vi "GetStartAndStopBlocks.vi"(8 "error in (no error)":errorcluster, 9 "data":T1) -> (0 "error out":errorcluster, 2 "stop block":T5, 3 "start block":T5)   [LabVIEW 2017, in "CmsDataEventCreator.lvlib"]
uses:
  <vilib>/addons/InsightCM/Devices/Shared/Cms/CmsDataEventCreator/CmsDataEventCreator.lvlib
  <vilib>/addons/InsightCM/Devices/Shared/Common/DVRBuffer/controls/BufferLocation.ctl
  <vilib>/addons/InsightCM/Devices/Shared/Common/DataFlow/controls/Data.ctl
  <vilib>/addons/InsightCM/Utilities/DataAccessors/controls/wfmSGL_DVR.ctl
  <vilib>/addons/PointValueMap/controls/PointMap.ctl
  <vilib>/addons/InsightCM/Devices/Shared/Common/DataFlow/controls/Type.ctl
  <vilib>/addons/PointValueMap/subVIs/Point_Read_variant.vi
  <vilib>/addons/PointValueMap/PointValueMap.lvlib
  <vilib>/addons/InsightCM/Devices/Shared/Common/DVRBuffer/DVRBuffer.lvlib
  <vilib>/addons/InsightCM/Devices/Shared/Common/DataFlow/DataFlow.lvlib
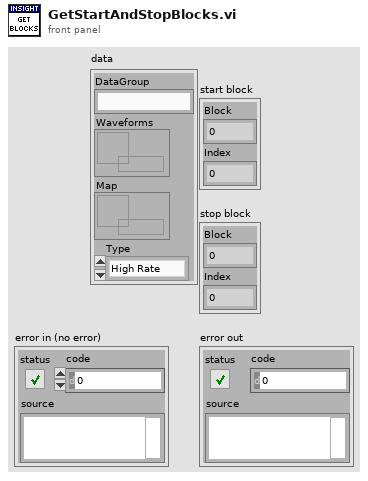
[diagram p1: front panel]
types:
  T1 = typedef "DataFlow.lvlib/Data.ctl" = cluster{"DataGroup":string, "Waveforms":T2, "Map":T3, "Type":T4}
  T2 = typedef "wfmSGL_DVR.ctl" = refnum<data-value>
  T3 = typedef "PointValueMap.lvlib/PointMap.ctl" = refnum<data-value>
  T4 = typedef "DataFlow.lvlib/Type.ctl" = enum16{"High Rate", "Low Rate", "Burst Mode"}
  T5 = typedef "DVRBuffer.lvlib/BufferLocation.ctl" = cluster{"Block":u32, "Index":i32}
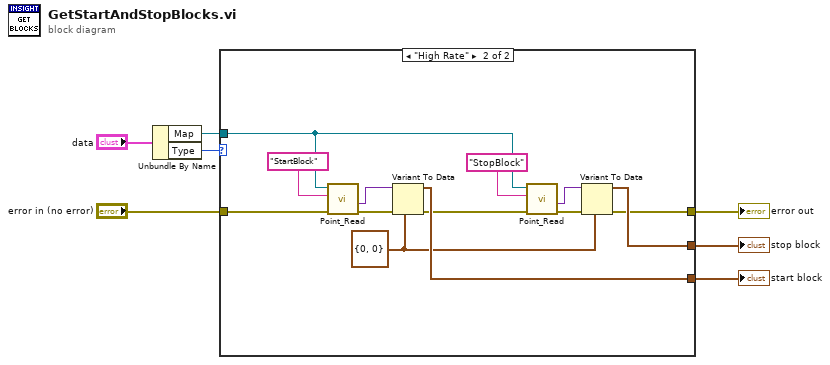
[diagram p0: block diagram]
diagram:
  n1 = Unbundle By Name("data") -> ("Map"=w2:T3, "Type"=w1:T4)
  n2 = case shown="\"High Rate\"" w1 {
    tunnel: [_ w21] -> w7
    tunnel: [_ w20] -> w6
    tunnel: "error in (no error)" -> [w8 w14]
    tunnel: [w8 w13] -> w4
    tunnel: w2 -> [_ w9]
    frame Default {
    }
    frame "High Rate" {
      w19 = T5 {"Block"=0, "Index"=0} ("buffer location")
      n3 = call-poly <vilib>:"Point_Read.vi"("Error In"=w14, "Tag"="StartBlock", "Map"=w9) -> ("Error Out"=w12:errorcluster, "Value"=w16:variant)  [unwired: 3 in, 4 out]
      n4 = Variant To Data(error in=w12, type=w19, Variant=w16) -> (data=w20:T5, error out=w11:errorcluster)
      n5 = call-poly <vilib>:"Point_Read.vi"("Error In"=w11, "Tag"="StopBlock", "Map"=w9) -> ("Error Out"=w10:errorcluster, "Value"=w17:variant)  [unwired: 3 in, 4 out]
      n6 = Variant To Data(error in=w10, type=w19, Variant=w17) -> (data=w21:T5, error out=w13:errorcluster)
    }
  }
  "stop block" <- w7
  "start block" <- w6
  "error out" <- w4
